vi "Memory Throughput Test PCIe-1473R (FPGA).vi"() -> ()   [LabVIEW 2013]
doc: "This test writes to and reads from external memory at maximum data rates and reports the total measured throughput. Varying the write and read grant time will directly affect the memory efficiency. The larger the grant time, then the larger the througput, and the lower the grant time, then the lower the throughput.\n\nDuring reads, the data is validated against an expected pattern. Failures will cause \"Read Data Error?\" to illuminate. To avoid read data errors, a full iteration of memory writes must be completed before starting the memory reads."
uses:
  <vilib>/Platform/TimedLoop/XDataNode/timing_clust.ctl
  <vilib>/Platform/TimedLoop/XDataNode/nitl_modes.ctl
  <vilib>/Platform/TimedLoop/XDataNode/wakeup.ctl
  DRAMElemReaderState.ctl
  Read Request Command.ctl
  <vilib>/rvi/Emulation/niFpgaSctlEmulationGetInTimedLoop.vi
  <vilib>/rvi/Emulation/niFpgaEmulationReportErrorSimple.vi
  <vilib>/rvi/Emulation/niFpgaGetClockAttributes.vi
  <vilib>/rvi/Emulation/niFpgaCriticalErrorInLSC.vi
  <vilib>/rvi/FIFO/Fifo_Resource/nirvififoEmulationWriteFpgaImpl.vi
  <vilib>/rvi/DataTransferAndStorage/Container/Common/niFpgaContainerGetUniqueNameForEmu.vi
  <vilib>/rvi/FIFO/Fifo_Resource/nirvififoEmulationReadFpgaImpl.vi
  <vilib>/rvi/Memory/Memory_Emulation/niFpgaMemoryEmulationReadFromVariant.vi
  <vilib>/rvi/Memory/Memory_Emulation/niFpgaMemoryFastEmulationDramWriteAndRequestData.vi
  <vilib>/rvi/Memory/Memory_Emulation/niFpgaMemoryEmulationDramWriteAndRequestData.vi
  <vilib>/rvi/Memory/Memory_Emulation/niFpgaMemoryEmulationWriteToVariant.vi
  <vilib>/Platform/TimedLoop/XDataNode/XDataNode.xnode
  <vilib>/rvi/DataTransferAndStorage/Container/XNode/niFpgaContainer.xnode
  <vilib>/rvi/FIFO/Fifo_Resource/nirvififoEmulationWrite.vi
  <vilib>/rvi/FIFO/Fifo_Resource/nirvififoEmulationRead.vi
  <vilib>/rvi/Memory/Memory_Emulation/niFpgaMemoryEmulationDramRetrieveData.vi
  <vilib>/Platform/TimedLoop/XDataNode/XDNodeRunTimeDep.lvlib
panel:
  in  "Write Req Grant Time (Bank 1)":u16=1000 caption="Write Req Grant Time (clocks)"
  in  "Read Req Grant Time (Bank 1)":u16=1000 caption="Read Req Grant Time (clocks)"
  in  "DRAM Size (elements) (Bank 0)":u32=8388608 caption="DRAM Size (elements)"
  in  "Read Req Grant Time (Bank 0)":u16=1000 caption="Read Req Grant Time (clocks)"
  in  "Write Req Grant Time (Bank 0)":u16=1000 caption="Write Req Grant Time (clocks)"
  out "Current Write Data (Bank 1)":u64 caption="Current Write Data" format="%.0x"
  out "Current Write Address (Bank 1)":u32 caption="Current Write Address" format="%.0x"
  in  "Enable Writes? (Bank 1)":bool caption="Enable Writes?"
  out "Write Throughput (bytes/sec) (Bank 1)":u32 caption="Write Throughput (bytes/sec)" format="%^.0e"
  out "Read FIFO Overflow? (Bank 1)":bool caption="Read FIFO Overflow?"
  out "Read Data Error? (Bank 1)":bool caption="Read Data Error?"
  out "Current Read Data (Bank 1)":u64 caption="Current Read Data" format="%.0x"
  out "Current Read Address (Bank 1)":u32 caption="Current Read Address" format="%.0x"
  in  "Enable Reads? (Bank 1)":bool caption="Enable Reads?"
  out "Read Throughput (bytes/sec) (Bank 1)":u32 caption="Read Throughput (bytes/sec)" format="%^.0e"
  in  "DRAM Size (elements) (Bank 1)":u32=8388608 caption="DRAM Size (elements)"
  out "Read Data Error? (Bank 0)":bool caption="Read Data Error?"
  out "Write Throughput (bytes/sec) (Bank 0)":u32 caption="Write Throughput (bytes/sec)" format="%^.0e"
  out "Read Throughput (bytes/sec) (Bank 0)":u32 caption="Read Throughput (bytes/sec)" format="%^.0e"
  in  "Enable Reads? (Bank 0)":bool caption="Enable Reads?"
  out "Read FIFO Overflow? (Bank 0)":bool caption="Read FIFO Overflow?"
  in  "Enable Writes? (Bank 0)":bool caption="Enable Writes?"
  out "Current Read Data (Bank 0)":u64 caption="Current Read Data" format="%.0x"
  out "Current Write Data (Bank 0)":u64 caption="Current Write Data" format="%.0x"
  out "Current Read Address (Bank 0)":u32 caption="Current Read Address" format="%.0x"
  out "Current Write Address (Bank 0)":u32 caption="Current Write Address" format="%.0x"
  # "Bank 0"
  # "Bank 1"
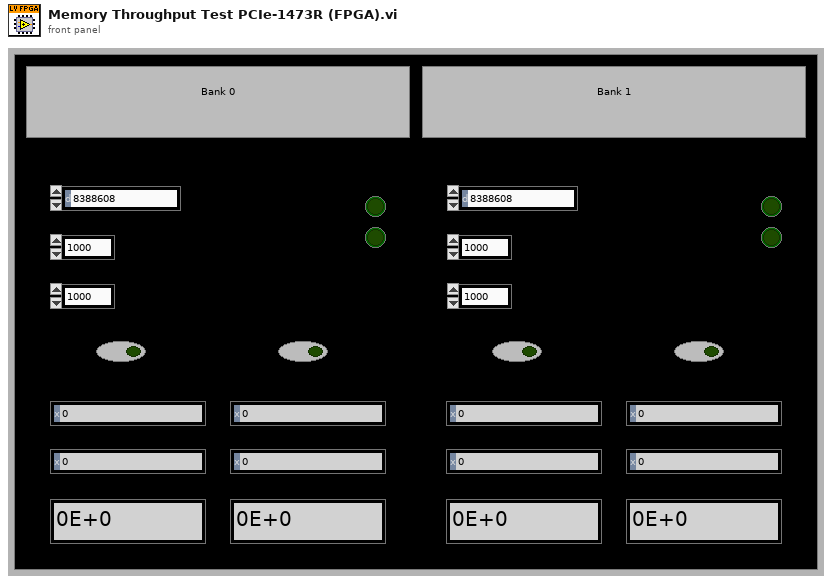
[diagram p1: front panel]
types:
  T1 = typedef "XDNodeRunTimeDep.lvlib/timing_clust.ctl" = cluster{"Expected End [f-1]":u64, "Actual End [f-1]":u64, "Finished Late? [f-1]":bool, "Expected End [i-1]":u64, "Actual End [i-1]":u64, "Finished Late? [i-1]":bool, "Expected Start [i]":u64, "Actual Start [i]":u64, "Expected Start [f]":u64, "Actual Start [f]":u64, "Source Name":string, "Structure Name":string, "Period":i64, "Deadline":i64, "Offset":i64, "Start":i64, "Priority":i32, "Timeout":i32, "Mode":T2, "Wakeup Reason":T3, "Error":errorcluster, "Source Type":string, "Secondary Source Type":string, "Global End Time":u64, "Global Start Time":u64, "Frame Duration":u64, "Iteration Duration":u64, "Assigned CPU":i32, "I/O Scan Engine Mode":u32}
  T2 = typedef "XDNodeRunTimeDep.lvlib/nitl_modes.ctl" = enum32{"No Change", "Process missed periods, maintain original phase", "Discard missed periods, maintain original phase", "Process missed periods, ignore original phase", "Discard missed periods, ignore original phase"}
  T3 = typedef "XDNodeRunTimeDep.lvlib/wakeup.ctl" = enum32{"Normal", "Aborted", "Asynchronous wakeup", "Timing source error", "Timed loop error", "Timeout"}
  T4 = typedef "DRAMElemReaderState.ctl" = enum16{"Start Read", "Wait for Read Complete"}
  T5 = typedef "Read Request Command.ctl" = cluster{"Address":u32, "Elements Remaining":u32, "Valid?":bool}
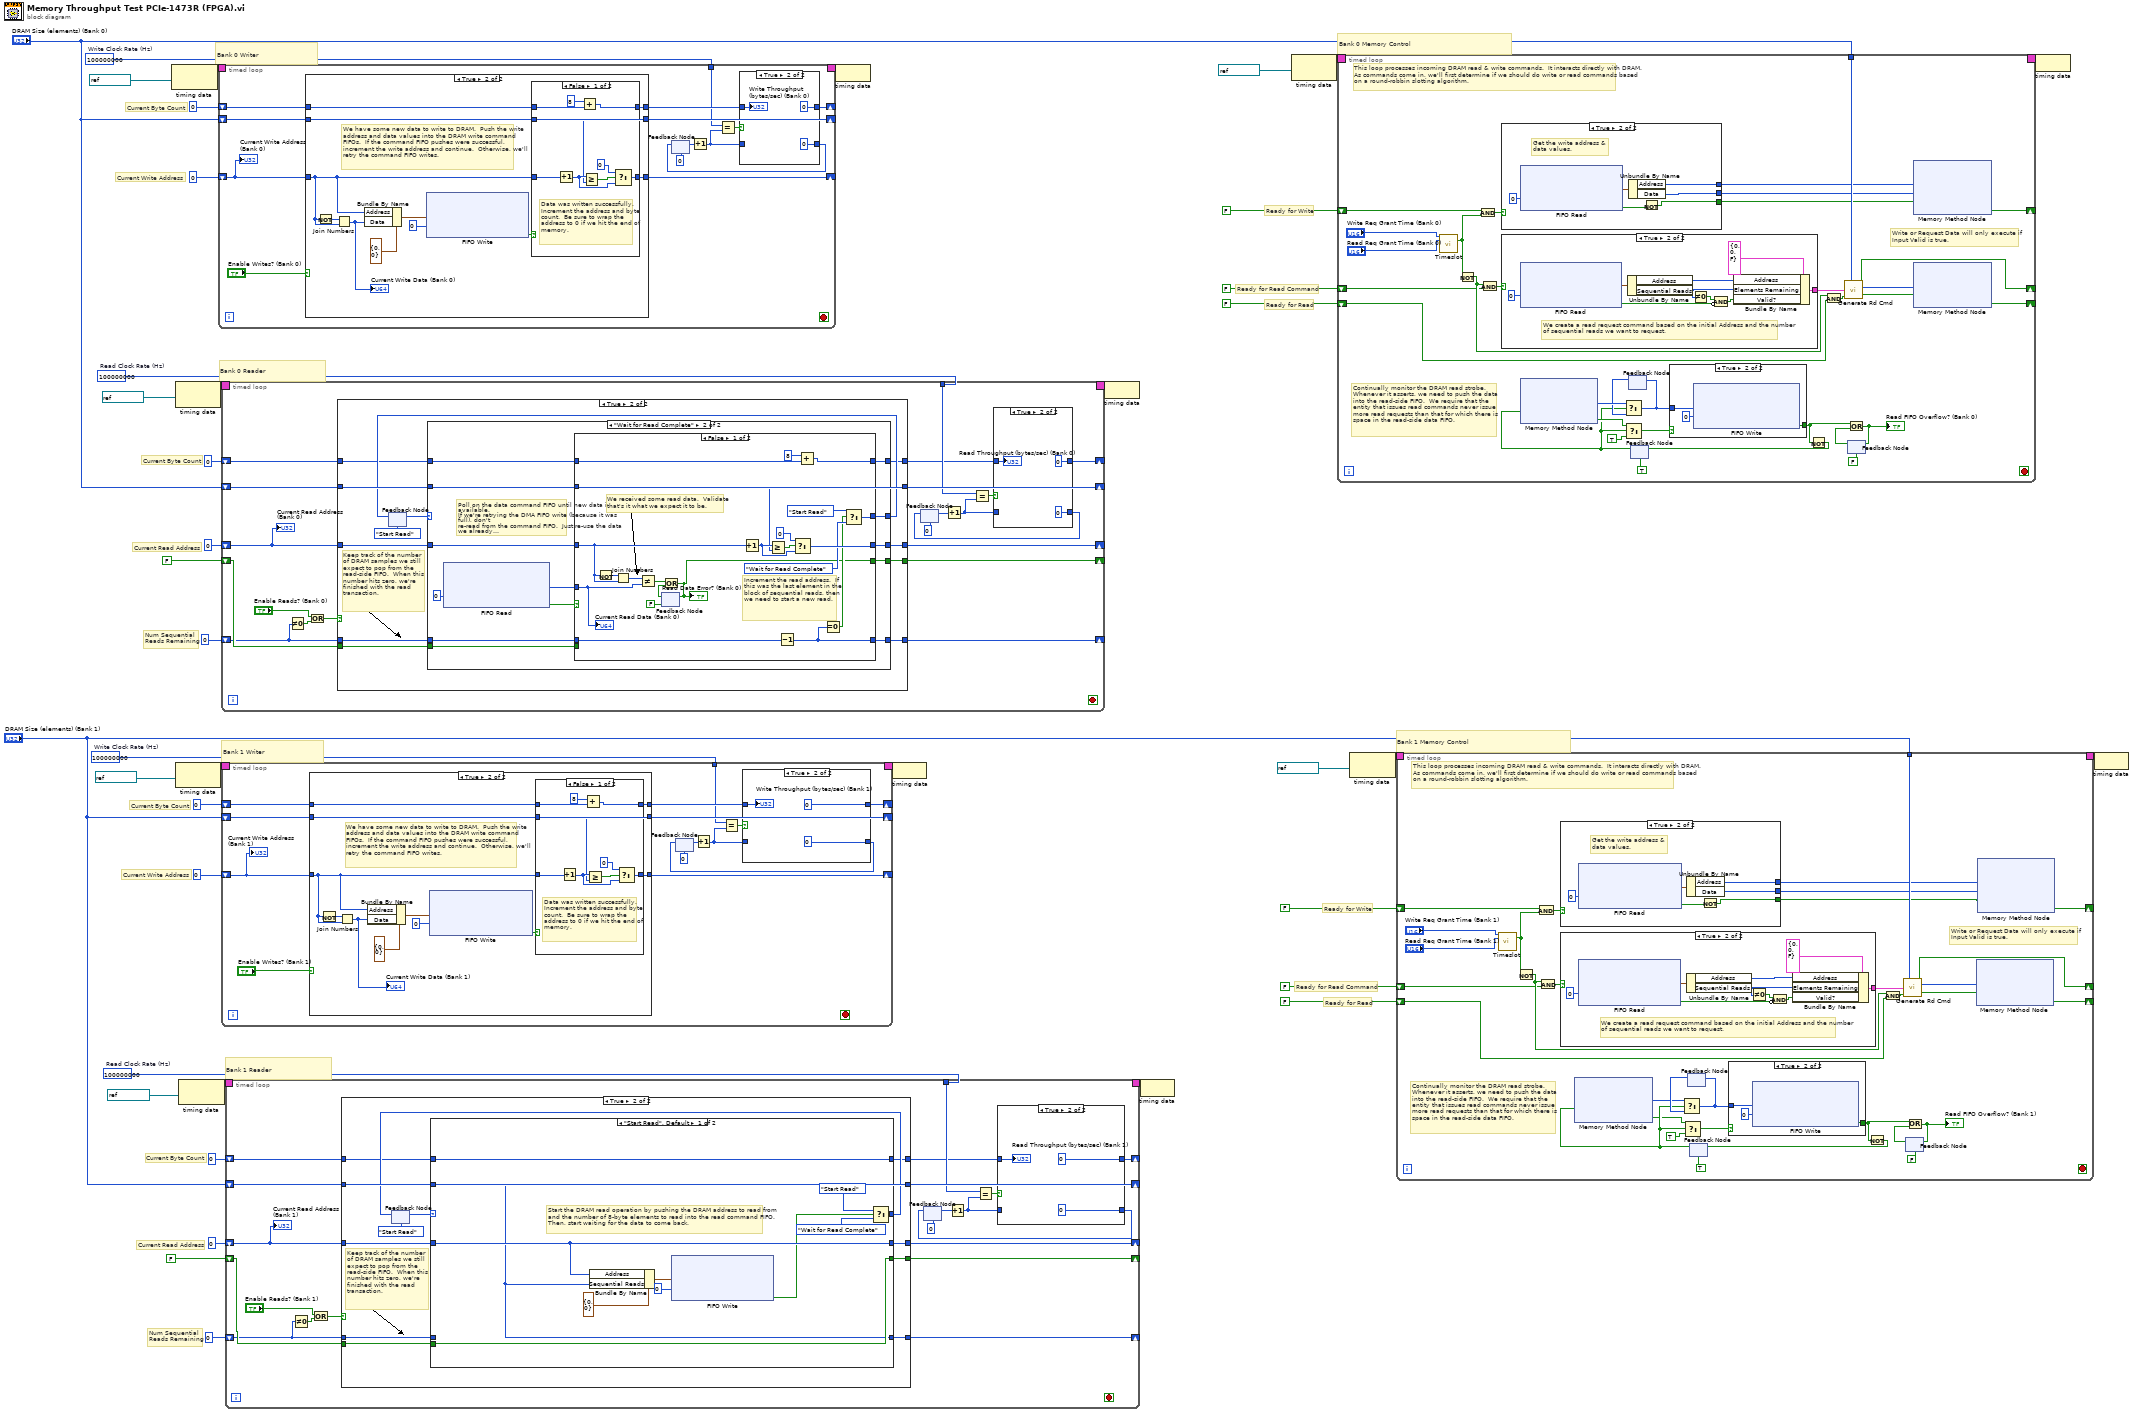
[diagram p0: block diagram]
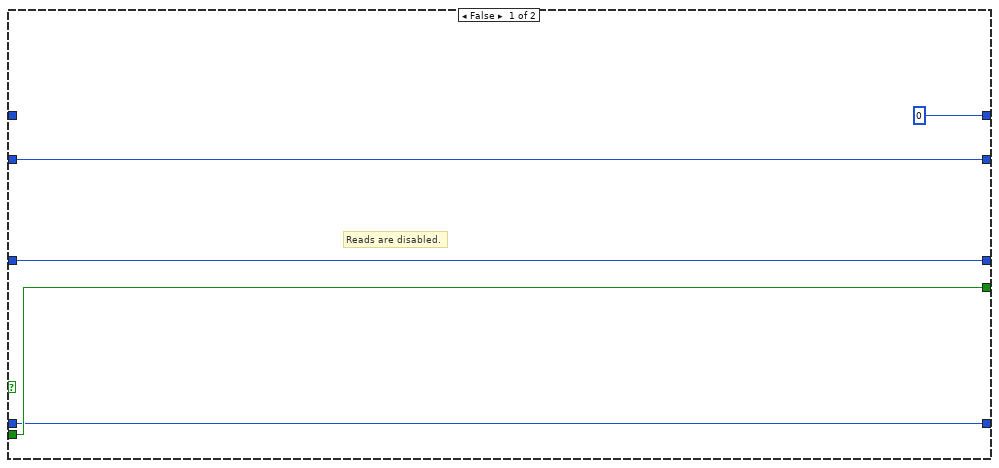
[diagram p3: hidden frame]
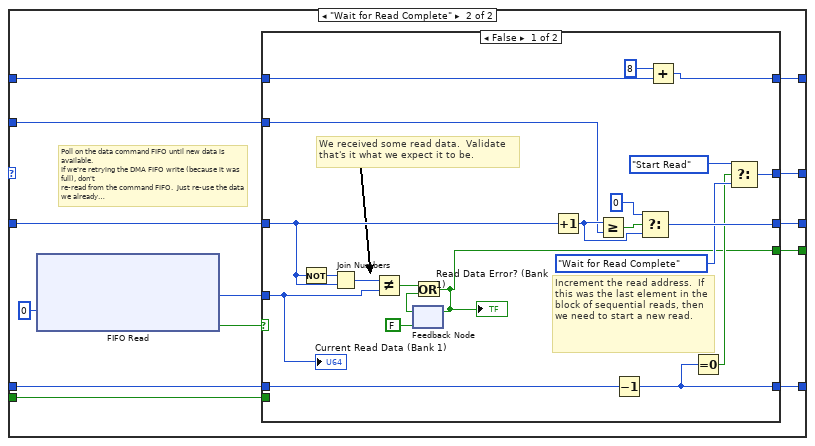
[diagram p4: hidden frame]
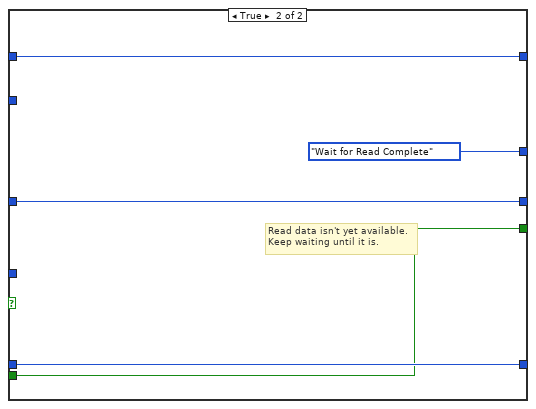
[diagram p5: hidden frame]
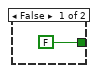
[diagram p6: hidden frame]
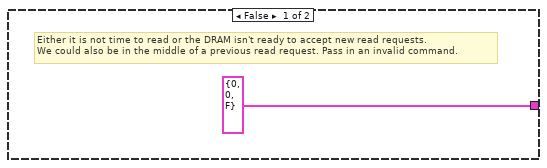
[diagram p7: hidden frame]
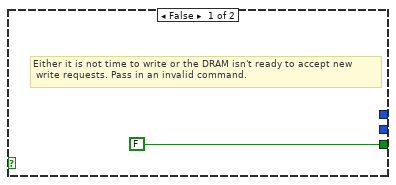
[diagram p8: hidden frame]
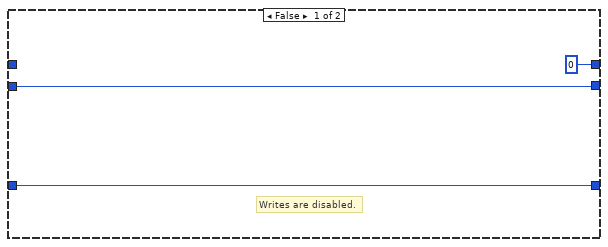
[diagram p10: hidden frame]
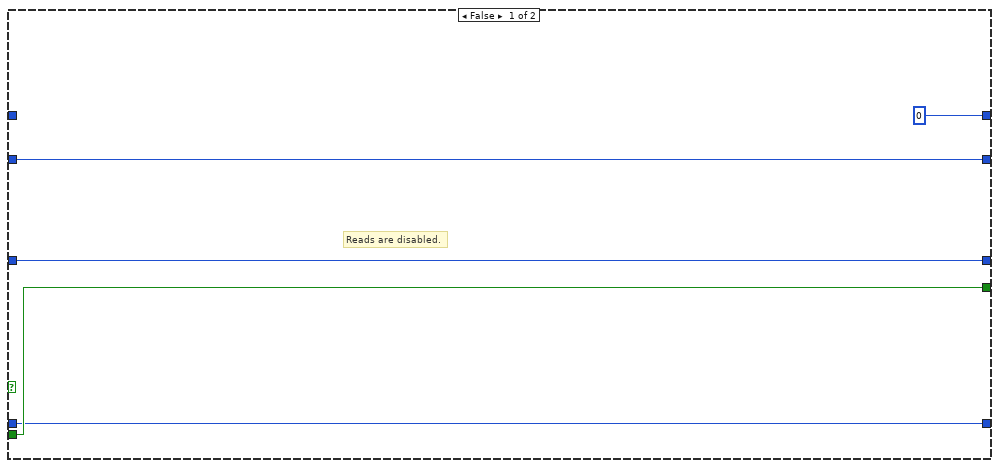
[diagram p13: hidden frame]
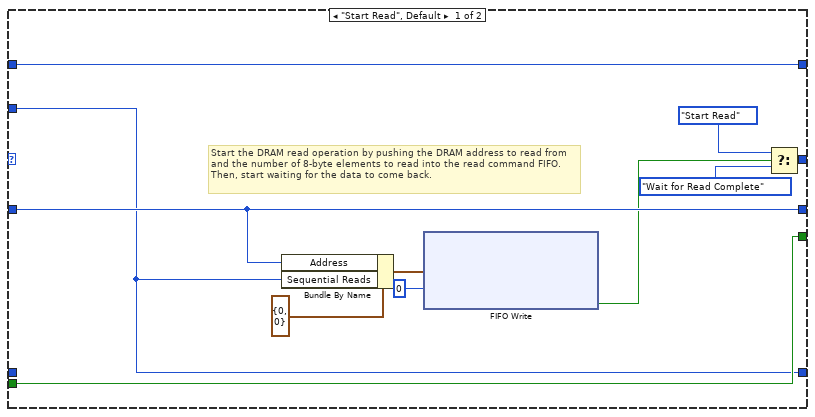
[diagram p14: hidden frame]
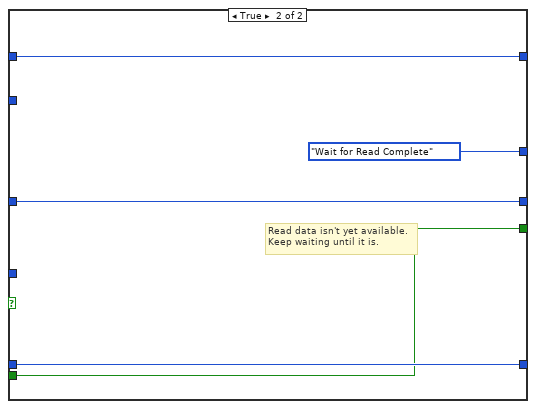
[diagram p15: hidden frame]
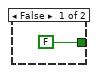
[diagram p16: hidden frame]
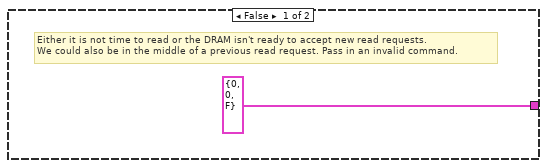
[diagram p17: hidden frame]
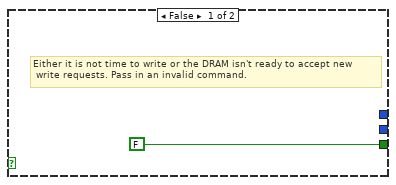
[diagram p18: hidden frame]
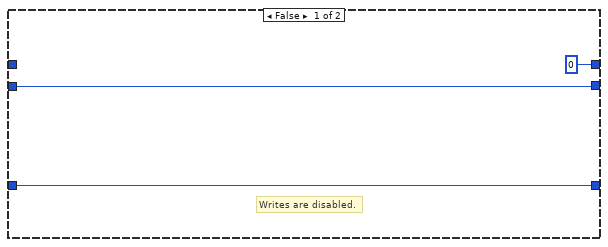
[diagram p20: hidden frame]
diagram:
  w2 = u32 100000000  # Read Clock Rate (Hz)
  w8 = u32 100000000  # Write Clock Rate (Hz)
  w28 = u32 100000000  # Read Clock Rate (Hz)
  w29 = u32 100000000  # Write Clock Rate (Hz)
  # "Ready for Read Command"
  # "Ready for Write"
  # "Ready for Read"
  # "Num Sequential\nReads Remaining"
  # "Bank 1 Memory Control"
  # "Bank 1 Reader"
  # "Bank 1 Writer"
  # "Current Byte Count"
  # "Current Byte Count"
  # "Current Read Address"
  # "Current Write Address"
  # "Ready for Read Command"
  # "Ready for Write"
  # "Ready for Read"
  # "Num Sequential\nReads Remaining"
  # "Bank 0 Memory Control"
  # "Bank 0 Reader"
  # "Bank 0 Writer"
  # "Current Byte Count"
  # "Current Byte Count"
  # "Current Read Address"
  # "Current Write Address"
  n1 = node-c288(refnum<k21> "100MHz" ("Source Name")) -> (w42:T1)
  n2 = node-c288(refnum<k21> "100MHz" ("Source Name")) -> (w38:T1)
  n3 = node-c288(refnum<k21> "100MHz" ("Source Name")) -> (w21:T1)
  n4 = node-c288(refnum<k21> "100MHz" ("Source Name")) -> (w17:T1)
  n5 = timed-loop {
    timing: w42 -> [_]
    timing-out: [_] -> w41
    shift-right: [w55] -> _
    shift-left: u32 0 -> [w56]
    shift-right: [w52] -> _
    shift-left: "DRAM Size (elements) (Bank 0)" -> [w54]
    shift-right: [w50] -> _
    shift-left: u32 0 -> [w51]
    tunnel: w29 -> [w43]
    stop <- _ stop-if-true
    n6 = case shown="True" "Enable Writes? (Bank 0)" {
      tunnel: w56 -> [w62 w69]
      tunnel: [w62 w75] -> w55
      tunnel: w54 -> [w63 w74]
      tunnel: [w63 w74] -> w52
      tunnel: w51 -> [_ w71]
      tunnel: [u32 0 w70] -> w49
      frame False {
        # "Writes are disabled."
      }
      frame True {
        # "We have some new data to write to DRAM.  Push the write address and data values into the DRAM write command FIFOs.  If the command FIFO pushes were successful, increment the write address and continue.  Otherwise, we'll retry the command FIFO writes."
        n7 = Not(x=w69) -> (.not. x?=w72:u32)
        n8 = Join Numbers(hi=w72, lo=w69) -> ((hi.lo)=w68:u64)
        "Current Write Data (Bank 0)" <- w68
        n9 = Bundle By Name(cluster=cluster{"Address":u32, "Data":u64} {"Address"=0, "Data"=0} ("Element"), "Address"=w69, "Data"=w68) -> (w66:cluster{"Address":u32, "Data":u64})
        n10 = xnode ("FIFO Write")("Element"=w66, "Timeout"=0) -> ("Timed Out?"=w67:bool)  [unwired: 1 in, 1 out]
        n11 = case shown="False" w67 {
          tunnel: w74 -> [w76 _]
          tunnel: [w81 w86] -> w75
          tunnel: w69 -> [w80 w86]
          tunnel: w71 -> [w79 w85]
          tunnel: [w77 w85] -> w70
          frame False {
            # "Data was written successfully.  Increment the address and byte count.  Be sure to wrap the address to 0 if we hit the end of memory."
            n12 = Increment(x=w80) -> (x+1=w82:u32)
            n13 = Add(x=u32 8, y=w79) -> (x+y=w77:u32)
            n14 = Greater Or Equal?(x=w82, y=w76) -> (x >= y?=w84:bool)
            n15 = Select(t=u32 0, s=w84, f=w82) -> (s? t:f=w81:u32)
          }
          frame True {
          }
        }
      }
    }
    n16 = feedback #1(u32 0) -> (w48:u32)
    n17 = Increment(x=w48) -> (x+1=w44:u32)
    n18 = Equal?(x=w43, y=w44) -> (x = y?=w46:bool)
    n19 = case shown="True" w46 {
      tunnel: w44 -> [w58 _]
      tunnel: [w58 u32 0] -> w45
      tunnel: w49 -> [w57 w59]
      tunnel: [w57 u32 0] -> w50
      frame False {
      }
      frame True {
        "Write Throughput (bytes/sec) (Bank 0)" <- w59
      }
    }
    n20 = feedback-in #1(w45) -> ()
    "Current Write Address (Bank 0)" <- w56
  }
  n21 = timed-loop {
    timing: w38 -> [_]
    timing-out: [_] -> w37
    shift-right: [w107] -> _
    shift-left: u32 0 -> [w108]
    shift-right: [w105] -> _
    shift-left: "DRAM Size (elements) (Bank 0)" -> [w106]
    shift-right: [w103] -> _
    shift-left: u32 0 -> [w104]
    tunnel: w28 -> [w102]
    shift-right: [w101] -> _
    shift-left: u32 0 -> [w91]
    shift-right: [w94] -> _
    shift-left: FALSE -> [w93]
    stop <- _ stop-if-true
    n22 = Not Equal To 0?(x=w91) -> (x != 0?=w92:bool)
    n23 = Or(x="Enable Reads? (Bank 0)", y=w92) -> (x .or. y?=w89:bool)
    n24 = case shown="True" w89 {
      tunnel: w108 -> [w116 w129]
      tunnel: [w116 w130] -> w107
      tunnel: w106 -> [w115 w128]
      tunnel: [w115 w128] -> w105
      tunnel: w104 -> [_ w124]
      tunnel: [u32 0 w123] -> w96
      tunnel: [w114 w122] -> w101
      tunnel: w91 -> [w114 w121]
      tunnel: [w117 w120] -> w94
      tunnel: w93 -> [w117 w119]
      frame False {
        # "Reads are disabled."
      }
      frame True {
        # "Keep track of the number\nof DRAM samples we still\nexpect to pop from the\nread-side FIFO.  When this\nnumber hits zero, we're\nfinished with the read\ntransaction."
        n25 = feedback #2(DRAMElemReaderState."Start Read") -> (w125:T4)
        n26 = case shown="\"Wait for Read Complete\"" w125 {
          tunnel: [w134 w153] -> w126
          tunnel: w129 -> [w137 w145]
          tunnel: [w137 w154] -> w130
          tunnel: w128 -> [w131 w151]
          tunnel: w121 -> [_ w149]
          tunnel: [w131 w150] -> w122
          tunnel: w124 -> [w140 w147]
          tunnel: [w140 w146] -> w123
          tunnel: [w133 w143] -> w120
          tunnel: w119 -> [w133 w142]
          frame "Start Read", Default {
            # "Start the DRAM read operation by pushing the DRAM address to read from and the number of 8-byte elements to read into the read command FIFO.  Then, start waiting for the data to come back."
            n27 = Bundle By Name(cluster=cluster{"Address":u32, "Sequential Reads":u32} {"Address"=0, "Sequential Reads"=0} ("Element"), "Address"=w137, "Sequential Reads"=w131) -> (w139:cluster{"Address":u32, "Sequential Reads":u32})
            n28 = xnode ("FIFO Write")("Element"=w139, "Timeout"=0) -> ("Timed Out?"=w136:bool)  [unwired: 1 in, 1 out]
            n29 = Select(t=DRAMElemReaderState."Start Read", s=w136, f=DRAMElemReaderState."Wait for Read Complete") -> (s? t:f=w134:T4)
          }
          frame "Wait for Read Complete" {
            # "Poll on the data command FIFO until new data is available.\nIf we're retrying the DMA FIFO write (because it was full), don't\nre-read from the command FIFO.  Just re-use the data we already\nread."
            n30 = xnode ("FIFO Read")("Timeout"=0) -> ("Element"=w144:u64, "Timed Out?"=w152:bool)  [unwired: 1 in, 1 out]
            n31 = case shown="False" w152 {
              tunnel: w145 -> [w163 w181]
              tunnel: [w175 w181] -> w154
              tunnel: [w176 DRAMElemReaderState."Wait for Read Complete"] -> w153
              tunnel: w144 -> [w157 _]
              tunnel: w151 -> [w161 _]
              tunnel: w149 -> [w174 w180]
              tunnel: [w160 w180] -> w150
              tunnel: w147 -> [w168 w179]
              tunnel: [w166 w179] -> w146
              tunnel: [w159 w177] -> w143
              tunnel: w142 -> [_ w177]
              frame False {
                # "Increment the read address.  If this was the last element in the block of sequential reads, then we need to start a new read."
                # "We received some read data.  Validate\nthat's it what we expect it to be."
                n32 = Not(x=w163) -> (.not. x?=w162:u32)
                n33 = Join Numbers(hi=w162, lo=w163) -> ((hi.lo)=w158:u64)
                n34 = Not Equal?(x=w158, y=w157) -> (x != y?=w156:bool)
                n35 = feedback #3(FALSE) -> (w165:bool)
                n36 = Or(x=w156, y=w165) -> (x .or. y?=w159:bool)
                "Read Data Error? (Bank 0)" <- w159
                n37 = feedback-in #3(w159) -> ()
                n38 = Increment(x=w163) -> (x+1=w172:u32)
                n39 = Greater Or Equal?(x=w172, y=w161) -> (x >= y?=w155:bool)
                n40 = Decrement(x=w174) -> (x-1=w160:u32)
                n41 = Select(t=u32 0, s=w155, f=w172) -> (s? t:f=w175:u32)
                n42 = Add(x=u32 8, y=w168) -> (x+y=w166:u32)
                n43 = Equal To 0?(x=w160) -> (x = 0?=w169:bool)
                n44 = Select(t=DRAMElemReaderState."Start Read", s=w169, f=DRAMElemReaderState."Wait for Read Complete") -> (s? t:f=w176:T4)
                "Current Read Data (Bank 0)" <- w157
              }
              frame True {
                # "Read data isn't yet available.\nKeep waiting until it is."
              }
            }
          }
        }
        n45 = feedback-in #2(w126) -> ()
      }
    }
    n46 = feedback #4(u32 0) -> (w99:u32)
    n47 = Increment(x=w99) -> (x+1=w97:u32)
    n48 = Equal?(x=w102, y=w97) -> (x = y?=w98:bool)
    n49 = case shown="True" w98 {
      tunnel: w97 -> [w110 _]
      tunnel: [w110 u32 0] -> w95
      tunnel: w96 -> [w109 w111]
      tunnel: [w109 u32 0] -> w103
      frame False {
      }
      frame True {
        "Read Throughput (bytes/sec) (Bank 0)" <- w111
      }
    }
    n50 = feedback-in #4(w95) -> ()
    "Current Read Address (Bank 0)" <- w108
  }
  n51 = timed-loop {
    timing: w21 -> [_]
    timing-out: [_] -> w20
    shift-right: [w197] -> _
    shift-left: u32 0 -> [w185]
    shift-right: [w195] -> _
    shift-left: "DRAM Size (elements) (Bank 1)" -> [w196]
    shift-right: [w193] -> _
    shift-left: u32 0 -> [w194]
    tunnel: w8 -> [w186]
    stop <- _ stop-if-true
    n52 = case shown="True" "Enable Writes? (Bank 1)" {
      tunnel: w185 -> [w203 w210]
      tunnel: [w203 w216] -> w197
      tunnel: w196 -> [w204 w215]
      tunnel: [w204 w215] -> w195
      tunnel: w194 -> [_ w212]
      tunnel: [u32 0 w211] -> w192
      frame False {
        # "Writes are disabled."
      }
      frame True {
        # "We have some new data to write to DRAM.  Push the write address and data values into the DRAM write command FIFOs.  If the command FIFO pushes were successful, increment the write address and continue.  Otherwise, we'll retry the command FIFO writes."
        n53 = Not(x=w210) -> (.not. x?=w213:u32)
        n54 = Join Numbers(hi=w213, lo=w210) -> ((hi.lo)=w206:u64)
        "Current Write Data (Bank 1)" <- w206
        n55 = Bundle By Name(cluster=cluster{"Address":u32, "Data":u64} {"Address"=0, "Data"=0} ("Element"), "Address"=w210, "Data"=w206) -> (w208:cluster{"Address":u32, "Data":u64})
        n56 = xnode ("FIFO Write")("Element"=w208, "Timeout"=0) -> ("Timed Out?"=w209:bool)  [unwired: 1 in, 1 out]
        n57 = case shown="False" w209 {
          tunnel: w215 -> [w217 _]
          tunnel: [w222 w227] -> w216
          tunnel: w210 -> [w221 w227]
          tunnel: w212 -> [w220 w226]
          tunnel: [w218 w226] -> w211
          frame False {
            # "Data was written successfully.  Increment the address and byte count.  Be sure to wrap the address to 0 if we hit the end of memory."
            n58 = Increment(x=w221) -> (x+1=w223:u32)
            n59 = Add(x=u32 8, y=w220) -> (x+y=w218:u32)
            n60 = Greater Or Equal?(x=w223, y=w217) -> (x >= y?=w225:bool)
            n61 = Select(t=u32 0, s=w225, f=w223) -> (s? t:f=w222:u32)
          }
          frame True {
          }
        }
      }
    }
    n62 = feedback #5(u32 0) -> (w191:u32)
    n63 = Increment(x=w191) -> (x+1=w187:u32)
    n64 = Equal?(x=w186, y=w187) -> (x = y?=w189:bool)
    n65 = case shown="True" w189 {
      tunnel: w187 -> [w199 _]
      tunnel: [w199 u32 0] -> w188
      tunnel: w192 -> [w198 w200]
      tunnel: [w198 u32 0] -> w193
      frame False {
      }
      frame True {
        "Write Throughput (bytes/sec) (Bank 1)" <- w200
      }
    }
    n66 = feedback-in #5(w188) -> ()
    "Current Write Address (Bank 1)" <- w185
  }
  n67 = timed-loop {
    timing: w17 -> [_]
    timing-out: [_] -> w16
    shift-right: [w249] -> _
    shift-left: u32 0 -> [w230]
    shift-right: [w247] -> _
    shift-left: "DRAM Size (elements) (Bank 1)" -> [w248]
    shift-right: [w245] -> _
    shift-left: u32 0 -> [w246]
    tunnel: w2 -> [w244]
    shift-right: [w243] -> _
    shift-left: u32 0 -> [w233]
    shift-right: [w236] -> _
    shift-left: FALSE -> [w235]
    stop <- _ stop-if-true
    n68 = Not Equal To 0?(x=w233) -> (x != 0?=w234:bool)
    n69 = Or(x="Enable Reads? (Bank 1)", y=w234) -> (x .or. y?=w232:bool)
    n70 = case shown="True" w232 {
      tunnel: w230 -> [w257 w270]
      tunnel: [w257 w271] -> w249
      tunnel: w248 -> [w256 w269]
      tunnel: [w256 w269] -> w247
      tunnel: w246 -> [_ w265]
      tunnel: [u32 0 w264] -> w238
      tunnel: [w255 w263] -> w243
      tunnel: w233 -> [w255 w262]
      tunnel: [w258 w261] -> w236
      tunnel: w235 -> [w258 w260]
      frame False {
        # "Reads are disabled."
      }
      frame True {
        # "Keep track of the number\nof DRAM samples we still\nexpect to pop from the\nread-side FIFO.  When this\nnumber hits zero, we're\nfinished with the read\ntransaction."
        n71 = feedback #6(DRAMElemReaderState."Start Read") -> (w266:T4)
        n72 = case shown="\"Start Read\", Default" w266 {
          tunnel: [w275 w294] -> w267
          tunnel: w270 -> [w278 w286]
          tunnel: [w278 w295] -> w271
          tunnel: w269 -> [w272 w292]
          tunnel: w262 -> [_ w290]
          tunnel: [w272 w291] -> w263
          tunnel: w265 -> [w281 w288]
          tunnel: [w281 w287] -> w264
          tunnel: [w274 w284] -> w261
          tunnel: w260 -> [w274 w283]
          frame "Start Read", Default {
            # "Start the DRAM read operation by pushing the DRAM address to read from and the number of 8-byte elements to read into the read command FIFO.  Then, start waiting for the data to come back."
            n73 = Bundle By Name(cluster=cluster{"Address":u32, "Sequential Reads":u32} {"Address"=0, "Sequential Reads"=0} ("Element"), "Address"=w278, "Sequential Reads"=w272) -> (w280:cluster{"Address":u32, "Sequential Reads":u32})
            n74 = xnode ("FIFO Write")("Element"=w280, "Timeout"=0) -> ("Timed Out?"=w277:bool)  [unwired: 1 in, 1 out]
            n75 = Select(t=DRAMElemReaderState."Start Read", s=w277, f=DRAMElemReaderState."Wait for Read Complete") -> (s? t:f=w275:T4)
          }
          frame "Wait for Read Complete" {
            # "Poll on the data command FIFO until new data is available.\nIf we're retrying the DMA FIFO write (because it was full), don't\nre-read from the command FIFO.  Just re-use the data we already\nread."
            n76 = xnode ("FIFO Read")("Timeout"=0) -> ("Element"=w285:u64, "Timed Out?"=w293:bool)  [unwired: 1 in, 1 out]
            n77 = case shown="False" w293 {
              tunnel: w286 -> [w304 w322]
              tunnel: [w316 w322] -> w295
              tunnel: [w317 DRAMElemReaderState."Wait for Read Complete"] -> w294
              tunnel: w285 -> [w297 _]
              tunnel: w292 -> [w302 _]
              tunnel: w290 -> [w315 w321]
              tunnel: [w301 w321] -> w291
              tunnel: w288 -> [w309 w320]
              tunnel: [w307 w320] -> w287
              tunnel: [w296 w318] -> w284
              tunnel: w283 -> [_ w318]
              frame False {
                # "Increment the read address.  If this was the last element in the block of sequential reads, then we need to start a new read."
                # "We received some read data.  Validate\nthat's it what we expect it to be."
                n78 = Not(x=w304) -> (.not. x?=w303:u32)
                n79 = Join Numbers(hi=w303, lo=w304) -> ((hi.lo)=w300:u64)
                n80 = Not Equal?(x=w300, y=w297) -> (x != y?=w299:bool)
                n81 = feedback #7(FALSE) -> (w306:bool)
                n82 = Or(x=w299, y=w306) -> (x .or. y?=w296:bool)
                "Read Data Error? (Bank 1)" <- w296
                n83 = feedback-in #7(w296) -> ()
                n84 = Increment(x=w304) -> (x+1=w313:u32)
                n85 = Greater Or Equal?(x=w313, y=w302) -> (x >= y?=w298:bool)
                n86 = Decrement(x=w315) -> (x-1=w301:u32)
                n87 = Select(t=u32 0, s=w298, f=w313) -> (s? t:f=w316:u32)
                n88 = Add(x=u32 8, y=w309) -> (x+y=w307:u32)
                n89 = Equal To 0?(x=w301) -> (x = 0?=w310:bool)
                n90 = Select(t=DRAMElemReaderState."Start Read", s=w310, f=DRAMElemReaderState."Wait for Read Complete") -> (s? t:f=w317:T4)
                "Current Read Data (Bank 1)" <- w297
              }
              frame True {
                # "Read data isn't yet available.\nKeep waiting until it is."
              }
            }
          }
        }
        n91 = feedback-in #6(w267) -> ()
      }
    }
    n92 = feedback #8(u32 0) -> (w241:u32)
    n93 = Increment(x=w241) -> (x+1=w239:u32)
    n94 = Equal?(x=w244, y=w239) -> (x = y?=w240:bool)
    n95 = case shown="True" w240 {
      tunnel: w239 -> [w251 _]
      tunnel: [w251 u32 0] -> w237
      tunnel: w238 -> [w250 w252]
      tunnel: [w250 u32 0] -> w245
      frame False {
      }
      frame True {
        "Read Throughput (bytes/sec) (Bank 1)" <- w252
      }
    }
    n96 = feedback-in #8(w237) -> ()
    "Current Read Address (Bank 1)" <- w230
  }
  n97 = node-c288(w41) -> ()
  n98 = node-c288(w20) -> ()
  n99 = node-c288(w37) -> ()
  n100 = node-c288(w16) -> ()
  n101 = node-c288(refnum<k21> "100MHz" ("Source Name")) -> (w40:T1)
  n102 = timed-loop {
    timing: w40 -> [_]
    timing-out: [_] -> w39
    tunnel: "DRAM Size (elements) (Bank 0)" -> [w345]
    shift-right: [w354] -> _
    shift-left: FALSE ("Ready for Input") -> [w325]
    shift-right: [w353] -> _
    shift-left: FALSE ("Ready for Input") -> [w349]
    shift-right: [w344] -> _
    shift-left: FALSE ("ready for input") -> [w341]
    stop <- _ stop-if-true
    # "Write or Request Data will only execute if \nInput Valid is true."
    # "Continually monitor the DRAM read strobe.\nWhenever it asserts, we need to push the data\ninto the read-side FIFO.  We require that the\nentity that issues read commands never issue\nmore read requests than that for which there is\nspace in the read-side data FIFO."
    # "This loop processes incoming DRAM read & write commands.  It interacts directly with DRAM.  \nAs commands come in, we'll first determine if we should do write or read commands based \non a round-robbin slotting algorithm."
    n103 = call "Timeslot.vi"("Write Req Grant Time (clocks)"="Write Req Grant Time (Bank 0)", "Read Req Grant Time (clocks)"="Read Req Grant Time (Bank 0)") -> ("Mux Select"=w348:bool)  [unwired: 13 in]
    n104 = Not(x=w348) -> (.not. x?=w342:bool)
    n105 = And(x=w349, y=w348) -> (x .and. y?=w350:bool)
    n106 = And(x=w342, y=w341) -> (x .and. y?=w347:bool)
    n107 = case shown="True" w350 {
      tunnel: [_ w375] -> w340
      tunnel: [_ w374] -> w339
      tunnel: [FALSE w373] -> w338
      frame False {
        # "Either it is not time to write or the DRAM isn't ready to accept new\n write requests. Pass in an invalid command."
      }
      frame True {
        # "Get the write address & data values."
        n108 = xnode ("FIFO Read")("Timeout"=0) -> ("Element"=w376:cluster{"Address":u32, "Data":u64}, "Timed Out?"=w377:bool)  [unwired: 1 in, 1 out]
        n109 = Unbundle By Name(w376) -> ("Address"=w375:u32, "Data"=w374:u64)
        n110 = Not(x=w377) -> (.not. x?=w373:bool)
      }
    }
    n111 = case shown="True" w347 {
      tunnel: [T5 {"Address"=0, "Elements Remaining"=0, "Valid?"=FALSE} ("Read request") w363] -> w346
      frame False {
        # "Either it is not time to read or the DRAM isn't ready to accept new read requests.\nWe could also be in the middle of a previous read request. Pass in an invalid command."
      }
      frame True {
        # "We create a read request command based on the initial Address and the number of sequential reads we want to request."
        n112 = xnode ("FIFO Read")("Timeout"=0) -> ("Element"=w369:cluster{"Address":u32, "Sequential Reads":u32}, "Timed Out?"=w367:bool)  [unwired: 1 in, 1 out]
        n113 = Unbundle By Name(w369) -> ("Address"=w368:u32, "Sequential Reads"=w366:u32)
        n114 = Not Equal To 0?(x=w366) -> (x != 0?=w370:bool)
        n115 = Compound Arithmetic op=AND(w370, invert w367) -> (w365:bool)
        n116 = Bundle By Name(cluster=T5 {"Address"=0, "Elements Remaining"=0, "Valid?"=FALSE} ("Read request"), "Address"=w368, "Elements Remaining"=w366, "Valid?"=w365) -> (w363:T5)
      }
    }
    n117 = feedback #9() -> (w334:u64)  [unwired: 1 in]
    n118 = feedback #10(TRUE) -> (w326:bool)
    n119 = xnode ("Memory Method Node")("Ready For Output"=w326) -> ("Data"=w335:u64, "Output Valid"=w329:bool)  [unwired: 1 in, 1 out]
    n120 = Select(t=w335, s=w326, f=w334) -> (s? t:f=w333:u64)
    n121 = Select(t=w329, s=w326, f=TRUE) -> (s? t:f=w328:bool)
    n122 = feedback-in #9(w333) -> ()
    n123 = case shown="True" w328 {
      tunnel: [FALSE ("Timed Out?") w360] -> w332
      tunnel: w333 -> [_ w359]
      frame False {
      }
      frame True {
        n124 = xnode ("FIFO Write")("Element"=w359, "Timeout"=0) -> ("Timed Out?"=w360:bool)  [unwired: 1 in, 1 out]
      }
    }
    n125 = Not(x=w332) -> (.not. x?=w331:bool)
    n126 = feedback-in #10(w331) -> ()
    n127 = And(x=w342, y=w325) -> (x .and. y?=w343:bool)
    n128 = call "Generate Rd Cmd.vi"("Number of Elements"=w345, "next Read request"=w346, "Ready for Read"=w343) -> ("ready for input"=w344:bool, "Address"=w337:u32, "Valid?"=w336:bool)  [unwired: 10 in]
    n129 = feedback #11(FALSE) -> (w356:bool)
    n130 = Or(x=w332, y=w356) -> (x .or. y?=w357:bool)
    "Read FIFO Overflow? (Bank 0)" <- w357
    n131 = feedback-in #11(w357) -> ()
    n132 = xnode ("Memory Method Node")("Address"=w340, "Data"=w339, "Input Valid"=w338) -> ("Ready For Input"=w353:bool)  [unwired: 1 in, 1 out]
    n133 = xnode ("Memory Method Node")("Address"=w337, "Input Valid"=w336) -> ("Ready For Input"=w354:bool)  [unwired: 1 in, 1 out]
  }
  n134 = node-c288(refnum<k21> "100MHz" ("Source Name")) -> (w19:T1)
  n135 = timed-loop {
    timing: w19 -> [_]
    timing-out: [_] -> w18
    tunnel: "DRAM Size (elements) (Bank 1)" -> [w404]
    shift-right: [w384] -> _
    shift-left: FALSE ("Ready for Input") -> [w392]
    shift-right: [w387] -> _
    shift-left: FALSE ("Ready for Input") -> [w408]
    shift-right: [w403] -> _
    shift-left: FALSE ("ready for input") -> [w400]
    stop <- _ stop-if-true
    # "Write or Request Data will only execute if \nInput Valid is true."
    # "Continually monitor the DRAM read strobe.\nWhenever it asserts, we need to push the data\ninto the read-side FIFO.  We require that the\nentity that issues read commands never issue\nmore read requests than that for which there is\nspace in the read-side data FIFO."
    # "This loop processes incoming DRAM read & write commands.  It interacts directly with DRAM.  \nAs commands come in, we'll first determine if we should do write or read commands based \non a round-robbin slotting algorithm."
    n136 = call "Timeslot.vi"("Write Req Grant Time (clocks)"="Write Req Grant Time (Bank 1)", "Read Req Grant Time (clocks)"="Read Req Grant Time (Bank 1)") -> ("Mux Select"=w407:bool)  [unwired: 13 in]
    n137 = Not(x=w407) -> (.not. x?=w401:bool)
    n138 = And(x=w408, y=w407) -> (x .and. y?=w409:bool)
    n139 = And(x=w401, y=w400) -> (x .and. y?=w406:bool)
    n140 = case shown="True" w409 {
      tunnel: [_ w431] -> w390
      tunnel: [_ w430] -> w389
      tunnel: [FALSE w429] -> w388
      frame False {
        # "Either it is not time to write or the DRAM isn't ready to accept new\n write requests. Pass in an invalid command."
      }
      frame True {
        # "Get the write address & data values."
        n141 = xnode ("FIFO Read")("Timeout"=0) -> ("Element"=w432:cluster{"Address":u32, "Data":u64}, "Timed Out?"=w433:bool)  [unwired: 1 in, 1 out]
        n142 = Unbundle By Name(w432) -> ("Address"=w431:u32, "Data"=w430:u64)
        n143 = Not(x=w433) -> (.not. x?=w429:bool)
      }
    }
    n144 = case shown="True" w406 {
      tunnel: [T5 {"Address"=0, "Elements Remaining"=0, "Valid?"=FALSE} ("Read request") w419] -> w405
      frame False {
        # "Either it is not time to read or the DRAM isn't ready to accept new read requests.\nWe could also be in the middle of a previous read request. Pass in an invalid command."
      }
      frame True {
        # "We create a read request command based on the initial Address and the number of sequential reads we want to request."
        n145 = xnode ("FIFO Read")("Timeout"=0) -> ("Element"=w425:cluster{"Address":u32, "Sequential Reads":u32}, "Timed Out?"=w423:bool)  [unwired: 1 in, 1 out]
        n146 = Unbundle By Name(w425) -> ("Address"=w424:u32, "Sequential Reads"=w422:u32)
        n147 = Not Equal To 0?(x=w422) -> (x != 0?=w426:bool)
        n148 = Compound Arithmetic op=AND(w426, invert w423) -> (w421:bool)
        n149 = Bundle By Name(cluster=T5 {"Address"=0, "Elements Remaining"=0, "Valid?"=FALSE} ("Read request"), "Address"=w424, "Elements Remaining"=w422, "Valid?"=w421) -> (w419:T5)
      }
    }
    n150 = feedback #12() -> (w399:u64)  [unwired: 1 in]
    n151 = feedback #13(TRUE) -> (w382:bool)
    n152 = xnode ("Memory Method Node")("Ready For Output"=w382) -> ("Data"=w383:u64, "Output Valid"=w381:bool)  [unwired: 1 in, 1 out]
    n153 = Select(t=w383, s=w382, f=w399) -> (s? t:f=w398:u64)
    n154 = Select(t=w381, s=w382, f=TRUE) -> (s? t:f=w394:bool)
    n155 = feedback-in #12(w398) -> ()
    n156 = case shown="True" w394 {
      tunnel: [FALSE ("Timed Out?") w416] -> w397
      tunnel: w398 -> [_ w415]
      frame False {
      }
      frame True {
        n157 = xnode ("FIFO Write")("Element"=w415, "Timeout"=0) -> ("Timed Out?"=w416:bool)  [unwired: 1 in, 1 out]
      }
    }
    n158 = Not(x=w397) -> (.not. x?=w396:bool)
    n159 = feedback-in #13(w396) -> ()
    n160 = And(x=w401, y=w392) -> (x .and. y?=w402:bool)
    n161 = call "Generate Rd Cmd.vi"("Number of Elements"=w404, "next Read request"=w405, "Ready for Read"=w402) -> ("ready for input"=w403:bool, "Address"=w386:u32, "Valid?"=w385:bool)  [unwired: 10 in]
    n162 = feedback #14(FALSE) -> (w413:bool)
    n163 = Or(x=w397, y=w413) -> (x .or. y?=w391:bool)
    "Read FIFO Overflow? (Bank 1)" <- w391
    n164 = feedback-in #14(w391) -> ()
    n165 = xnode ("Memory Method Node")("Address"=w386, "Input Valid"=w385) -> ("Ready For Input"=w384:bool)  [unwired: 1 in, 1 out]
    n166 = xnode ("Memory Method Node")("Address"=w390, "Data"=w389, "Input Valid"=w388) -> ("Ready For Input"=w387:bool)  [unwired: 1 in, 1 out]
  }
  n167 = node-c288(w39) -> ()
  n168 = node-c288(w18) -> ()
